vi "Uploading Audio File to ELVIS.vi"(2 "Message":string, 8 "error in (no error)":errorcluster, 9 "Host ID":string="172.22.11.2", 10 "New File Name":string="Audio", 11 "Music File":path) -> (0 "error out":errorcluster)   [LabVIEW 2019]
doc: "This VI converts a Music file to a readable NI ELVIS III file. After making the convertion, the file is saved into the projects folder and then transfered to the target's media folder."
uses:
  <vilib>/Platform/storage/lvStorage.llb/_openFunction.ctl
  <vilib>/Platform/storage/lvStorage.llb/_openStorageWithRootAutoDetect.vi
  <vilib>/Platform/storage/lvStorage.llb/xStorage/xStorageSupp/ErrorOut.vi
  <vilib>/Platform/storage/lvStorage.llb/_queryPropPoly.vi
  <vilib>/Platform/storage/lvStorage.llb/_queryPropString.vi
  <vilib>/Platform/storage/lvStorage.llb/_queryGenericObjects.vi
  <vilib>/Platform/storage/lvStorage.llb/_loadAllDouble.vi
  Uploading to ELVIS Global Variables.vi
  <vilib>/Platform/storage/lvStorage.llb/xStorage/Open Data Storage/Open Data Storage.xnode
  <vilib>/Platform/storage/lvStorage.llb/xStorage/Read Data/Read Data.xnode
  <vilib>/FTP/NI_FTP.lvlib
panel:
  out "Signal Out":dbl(graph) caption="Audio Signal Out"
  # "Creating and Uploading an Audio File into a NI ELVIS III"
  # "This VI converts a Music file to a readable NI ELVIS III file. After making the convertion, the file is saved into the projects folder and then transfered to the target's media folder.\n\nRemember to use this VI for transfering the music or audio file before running any of the Audio VIs on the equipment.\n\nThe data tranference might take a while. Please, do not abort the VI or disconnect the target while this VI is running."
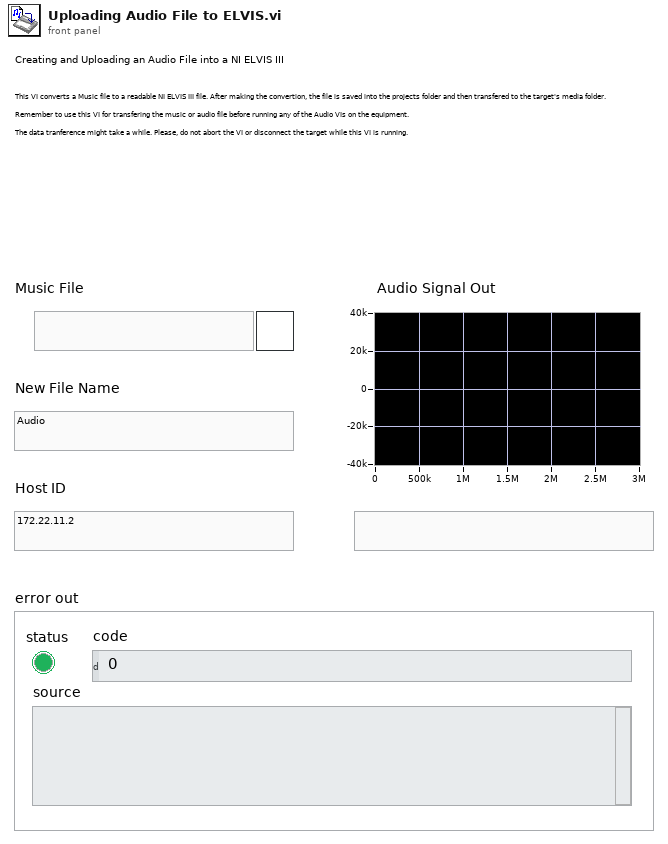
[diagram p1: front panel]
types:
  T1 = enum16{"open", "replace", "create", "open or create", "replace or create", "replace or create with confirmation"}
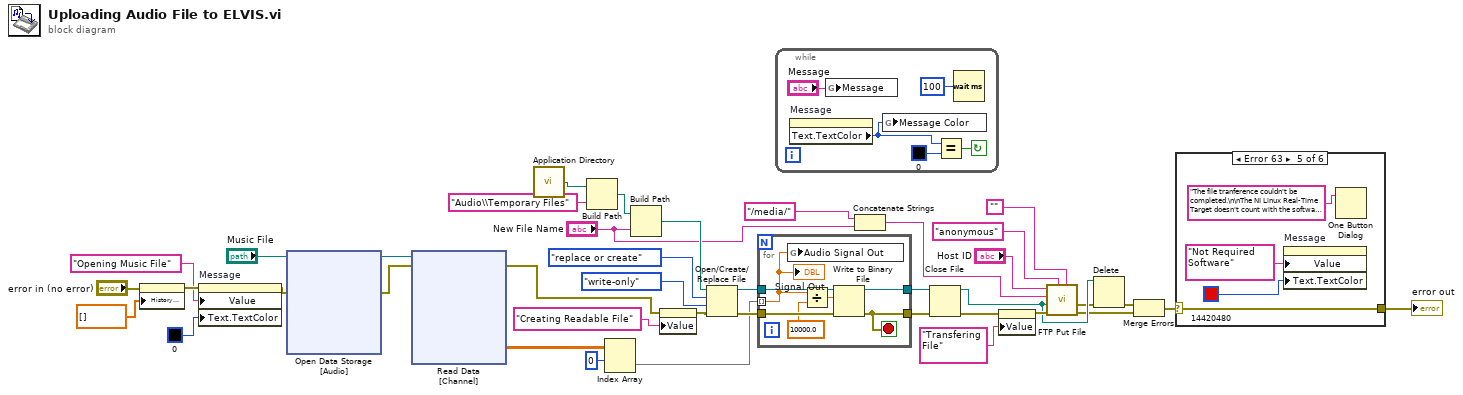
[diagram p0: block diagram]
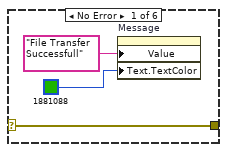
[diagram p2: hidden frame]
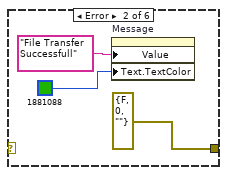
[diagram p3: hidden frame]
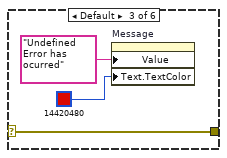
[diagram p4: hidden frame]
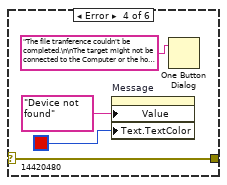
[diagram p5: hidden frame]
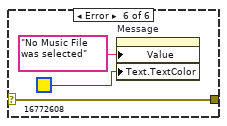
[diagram p6: hidden frame]
diagram:
  n1 = property on="Signal Out" class="WFChart (strict)"(error in="error in (no error)", "History Data"=dbl[] []) -> (error out=w22:errorcluster)  [unwired: 1 in, 1 out]
  n2 = property on="Message" class="Str"(error in=w22, "Value"="Opening Music File" ("Message"), "Text.TextColor"=u32 0 ("Text.Text Colors:Text Color")) -> (error out=w21:errorcluster)  [unwired: 1 in, 1 out]
  n3 = xnode "Open Data Storage\n[Audio]"("file path"="Music File", "error in (no error)"=w21) -> ("storage refnum (file)"=w38:refnum<k20>, "error out"=w39:errorcluster)  [unwired: 3 in, 1 out]
  n4 = xnode "Read Data\n[Channel]"("storage refnum (file)"=w38, "error in"=w39) -> ("Signal"=w37:dbl[][], "error out"=w18:errorcluster)  [unwired: 2 in, 2 out]
  n5 = call <vilib>:"Application Directory.vi"() -> ("Application Directory"=w8:path)
  n6 = Build Path(base path=w8, name or relative path="Audio\\Temporary Files") -> (appended path=w9:path)
  n7 = Index Array(array=w37, index (row)=0) -> (element=w26:dbl[])  [unwired: 1 in]
  n8 = Build Path(base path=w9, name or relative path="New File Name") -> (appended path=w27:path)
  n9 = property on="Message" class="Str"(error in=w18, "Value"="Creating Readable File" ("Message")) -> (error out=w19:errorcluster)  [unwired: 1 in, 1 out]
  n10 = Open/Create/Replace File(file path (use dialog)=w27, error in=w19, operation (0:open)=T1."replace or create", access (0:read/write)=enum16{"read/write", "read-only", "write-only"}."write-only") -> (refnum out=w35:refnum<file>, error out=w34:errorcluster)  [unwired: 2 in, 1 out]
  n11 = for {
    tunnel: w26 -> [w43] mode=indexing
    tunnel: w35 -> [w47]
    tunnel: [w45] -> w33
    tunnel: w34 -> [w46]
    tunnel: [w44] -> w32
    stop <- w44 stop-if-true
    n12 = global write "Uploading to ELVIS Global Variables.vi" "Audio Signal Out"(w43) -> ()
    n13 = Divide(x=w43, y=10000.0) -> (x/y=w42:dbl)
    n14 = Write to Binary File(file (use dialog)=w47, data=w42, error in=w46) -> (refnum out=w45:refnum<file>, error out=w44:errorcluster)  [unwired: 3 in, 1 out]
    "Signal Out" <- w43
  }
  n15 = while {
    stop <- w51 continue-if-true
    n16 = property on="Message" class="Str"() -> ("Text.TextColor"=w49:u32)  [unwired: 2 in, 2 out]
    n17 = global write "Uploading to ELVIS Global Variables.vi" "Message"("Message") -> ()
    n18 = global write "Uploading to ELVIS Global Variables.vi" "Message Color"(w49) -> ()
    n19 = Equal?(x=w49, y=u32 0 ("Text.Text Colors:Text Color")) -> (x = y?=w51:bool)
    n20 = Wait (ms)(milliseconds to wait=u32 100) -> ()  [unwired: 1 out]
  }
  n21 = Concatenate Strings("/media/", "New File Name") -> (w12:string)
  n22 = Close File(refnum=w33, error in=w32) -> (path=w10:path, error out=w15:errorcluster)
  n23 = property on="Message" class="Str"(error in=w15, "Value"="Transfering File" ("Message")) -> (error out=w14:errorcluster)  [unwired: 1 in, 1 out]
  n24 = call <vilib>:"FTP Put File.vi"("password"="", "user"="anonymous", "error in (no error)"=w14, "local path"=w10, "remote path"=w12, "host"="Host ID") -> ("error out"=w3:errorcluster, "file error"=w4:errorcluster)  [unwired: 4 in]
  n25 = Delete(path (use dialog)=w10, error in=w4) -> (error out=w2:errorcluster)  [unwired: 3 in, 2 out]
  n26 = Merge Errors(w2, w3) -> (w1:errorcluster)
  n27 = case shown="Error 63" w1 {
    selector: w1 -> [w53 _ w59 w62 w66 w70]
    tunnel: [w53 errorcluster {"status"=FALSE, "code"=0, "source"=""} ("error IO") w59 w62 w66 w70] -> w25
    frame No Error {
      n28 = property on="Message" class="Str"("Value"="File Transfer Successfull" ("Message"), "Text.TextColor"=u32 1881088 ("Text.Text Colors:Text Color")) -> ()  [unwired: 2 in, 2 out]
    }
    frame Error {
      n29 = property on="Message" class="Str"("Value"="File Transfer Successfull" ("Message"), "Text.TextColor"=u32 1881088 ("Text.Text Colors:Text Color")) -> ()  [unwired: 2 in, 2 out]
    }
    frame Default {
      n30 = property on="Message" class="Str"("Value"="Undefined Error has ocurred" ("Message"), "Text.TextColor"=u32 14420480 ("Text.Text Colors:Text Color")) -> ()  [unwired: 2 in, 2 out]
    }
    frame Error {
      n31 = property on="Message" class="Str"("Value"="Device not found" ("Message"), "Text.TextColor"=u32 14420480 ("Text.Text Colors:Text Color")) -> ()  [unwired: 2 in, 2 out]
      n32 = One Button Dialog(message="The file tranference couldn't be completed.\n\nThe target might not be connected to the Computer or the host ID is incorrect.\n\nVerify that the target is turned on and connected correctly. Once done this, check that the Host ID from the equipment corresponds to the Host ID control.") -> ()  [unwired: 1 in, 1 out]
    }
    frame Error {
      n33 = property on="Message" class="Str"("Value"="Not Required Software" ("Message"), "Text.TextColor"=u32 14420480 ("Text.Text Colors:Text Color")) -> ()  [unwired: 2 in, 2 out]
      n34 = One Button Dialog(message="The file tranference couldn't be completed.\n\nThe NI Linux Real-Time Target doesn't count with the software for file transference.\n\nTo allow file transference between devices look for  \"Using FTP With an NI Linux Real-Time Target\" in the following link and follow its instructions.\n\nhttps://knowledge.ni.com/") -> ()  [unwired: 1 in, 1 out]
    }
    frame Error {
      n35 = property on="Message" class="Str"("Value"="No Music File was selected" ("Message"), "Text.TextColor"=u32 16772608 ("Text.Text Colors:Text Color")) -> ()  [unwired: 2 in, 2 out]
    }
  }
  "error out" <- w25
